vi "Re-InitializaPlots.vi"(8 "error in (no error)":errorcluster, 10 "Cluster Of Graphs":T1) -> (0 "error out":errorcluster)   [LabVIEW 2015]
uses:
  TypeDef/GraphReff.ctl
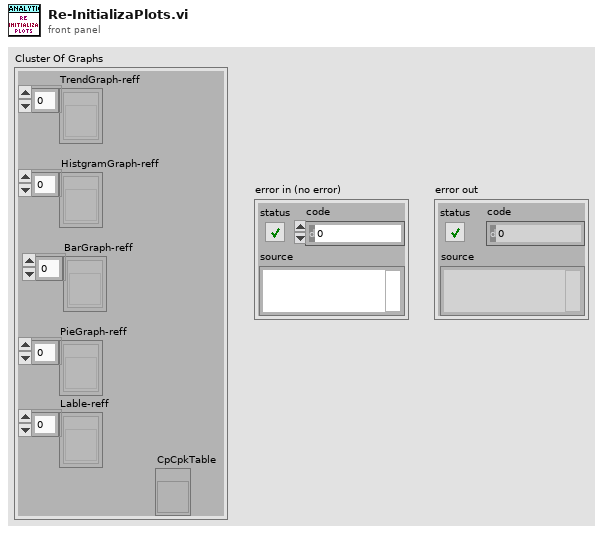
[diagram p1: front panel]
types:
  T1 = typedef "GraphReff.ctl" = cluster{"HistgramGraph-reff":refnum<vi>[], "BarGraph-reff":refnum<vi>[], "PieGraph-reff":refnum<vi>[], "Lable-reff":refnum<vi>[], "TrendGraph-reff":refnum<vi>[], "CpCpkTable":refnum<vi>}
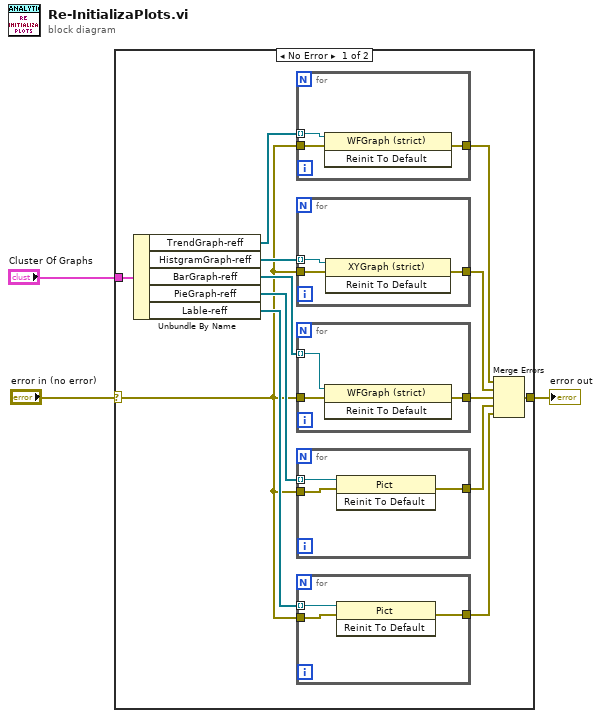
[diagram p0: block diagram]
diagram:
  n1 = case shown="No Error" "error in (no error)" {
    selector: "error in (no error)" -> [w10 w32]
    tunnel: "Cluster Of Graphs" -> [w16 _]
    tunnel: [w4 w32] -> w1
    frame No Error {
      n2 = Unbundle By Name(w16) -> ("TrendGraph-reff"=w15:refnum<vi>[], "HistgramGraph-reff"=w14:refnum<vi>[], "BarGraph-reff"=w13:refnum<vi>[], "PieGraph-reff"=w12:refnum<vi>[], "Lable-reff"=w11:refnum<vi>[])
      n3 = for {
        tunnel: w15 -> [w31] mode=indexing
        tunnel: w10 -> [w30]
        tunnel: [w29] -> w9
        n4 = invoke class="WFGraph (strict)" method="Reinit To Default"(reference=w31, error in=w30) -> (error out=w29:errorcluster)  [unwired: 1 in, 2 out]
      }
      n5 = for {
        tunnel: w14 -> [w28] mode=indexing
        tunnel: w10 -> [w27]
        tunnel: [w26] -> w8
        n6 = invoke class="XYGraph (strict)" method="Reinit To Default"(reference=w28, error in=w27) -> (error out=w26:errorcluster)  [unwired: 1 in, 2 out]
      }
      n7 = for {
        tunnel: w13 -> [w25] mode=indexing
        tunnel: w10 -> [w24]
        tunnel: [w23] -> w7
        n8 = invoke class="WFGraph (strict)" method="Reinit To Default"(reference=w25, error in=w24) -> (error out=w23:errorcluster)  [unwired: 1 in, 2 out]
      }
      n9 = for {
        tunnel: w12 -> [w22] mode=indexing
        tunnel: w10 -> [w21]
        tunnel: [w20] -> w6
        n10 = invoke class="Pict" method="Reinit To Default"(reference=w22, error in=w21) -> (error out=w20:errorcluster)  [unwired: 1 in, 2 out]
      }
      n11 = for {
        tunnel: w11 -> [w19] mode=indexing
        tunnel: w10 -> [w18]
        tunnel: [w17] -> w5
        n12 = invoke class="Pict" method="Reinit To Default"(reference=w19, error in=w18) -> (error out=w17:errorcluster)  [unwired: 1 in, 2 out]
      }
      n13 = Merge Errors(w9, w8, w7, w6, w5) -> (w4:errorcluster)
    }
    frame Error {
    }
  }
  "error out" <- w1
